vi "Arduino_RTTTL.vi"() -> ()   [LabVIEW 2011]
uses:
  <vilib>/LabVIEW Interface for Arduino/LabVIEW Interface for Arduino.lvlib
panel:
  in  "Insert RTTTL":string
  out "Parsed Song":T1
  in  "stop":bool
  # "Default duration"
  # "Default octave"
  # "Beat"
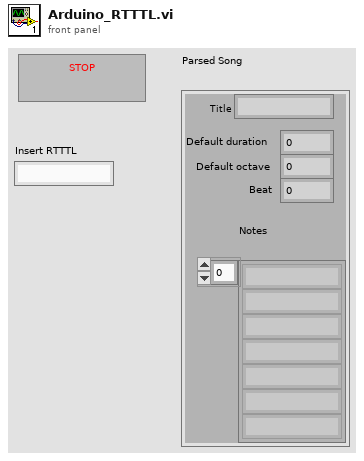
[diagram p1: front panel]
types:
  T1 = cluster{"Title":string, i32, i32, i32, "Notes":string[]}
  T2 = cluster{string, i32, i32, i32, "array type (1D String)":string[]}
  T3 = typedef "LabVIEW Interface for Arduino.lvlib/Arduino Resource.ctl" = cluster{"VISA resource":refnum<visa-resource-name>, "Board Type":T4, "Connection Type":enum8{"USB / Serial"}, "Bytes Per Packet (15)":u8}
  T4 = typedef "LabVIEW Interface for Arduino.lvlib/Board Type.ctl" = enum16{"Uno", "Dimuelanove w/Atmega 328", "Mega 2560"}
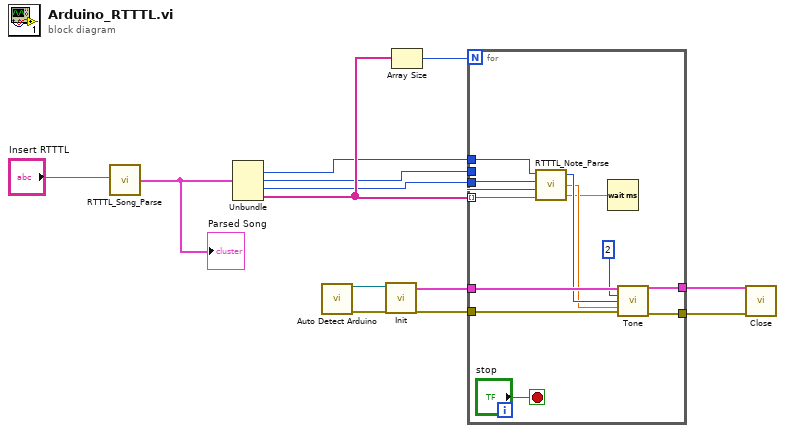
[diagram p0: block diagram]
diagram:
  n1 = call "RTTTL_Song_Parse.vi"("String"="Insert RTTTL") -> ("Cluster"=w7:T2)
  "Parsed Song" <- w7
  n2 = Unbundle(w7) -> (w4:i32, w3:i32, w2:i32, "array type (1D String)"=w5:string[])  [unwired: 1 out]
  n3 = call <vilib>:"Auto Detect Arduino.vi"() -> ("VISA resource"=w12:refnum<visa-resource-name>, "error out"=w13:errorcluster)  [unwired: 14 in]
  n4 = call <vilib>:"Init.vi"("VISA resource"=w12, "error in"=w13) -> ("Arduino Resource"=w10:T3, "error out"=w11:errorcluster)  [unwired: 16 in]
  n5 = Array Size(array=w5) -> (size(s)=w6:i32)
  n6 = for {
    N: w6 -> [_]
    tunnel: w11 -> [w26]
    tunnel: [w25] -> w9
    tunnel: [w24] -> w8
    tunnel: w10 -> [w23]
    tunnel: w5 -> [w20] mode=indexing
    tunnel: w4 -> [w19]
    tunnel: w3 -> [w18]
    tunnel: w2 -> [w17]
    stop <- "stop" stop-if-true
    n7 = call "RTTTL_Note_Parse.vi"("Element"=w20, "Beat"=w17, "Default octave"=w18, "Default duration"=w19) -> ("Pause"=w14:dbl, "Duration"=w15:dbl, "Frequency"=w16:i32)
    n8 = Wait (ms)(milliseconds to wait=w14) -> ()  [unwired: 1 out]
    n9 = call <vilib>:"Tone.vi"("Arduino Resource"=w23, "Tone DO Pin"=u8 2, "Frequency (0 Hz)"=w16, "Duration (1 ms)"=w15, "error in"=w26) -> ("Arduino Resource"=w24:T3, "error out"=w25:errorcluster)  [unwired: 9 in]
  }
  n10 = call <vilib>:"Close.vi"("Arduino Resource"=w8, "error in"=w9) -> ()  [unwired: 13 in, 1 out]
